vi "motor speed.vi"(0 "IN_A":refnum<k21>="ConnectorA/DIO2", 1 "IN_B":refnum<k21>="ConnectorA/DIO0", 2 "Enable":refnum<k21>="ConnectorA/DIO1", 3 "PWM":refnum<k21>="ConnectorA/DIO8", 4 "speed":i64, 5 "periode":i64, 6 "enable divider":bool, 7 "divider":fxp<+,4,4>, 9 "brake":bool) -> ()   [LabVIEW 2019]
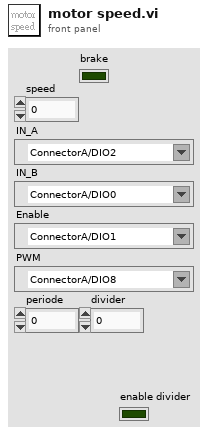
[diagram p1: front panel]
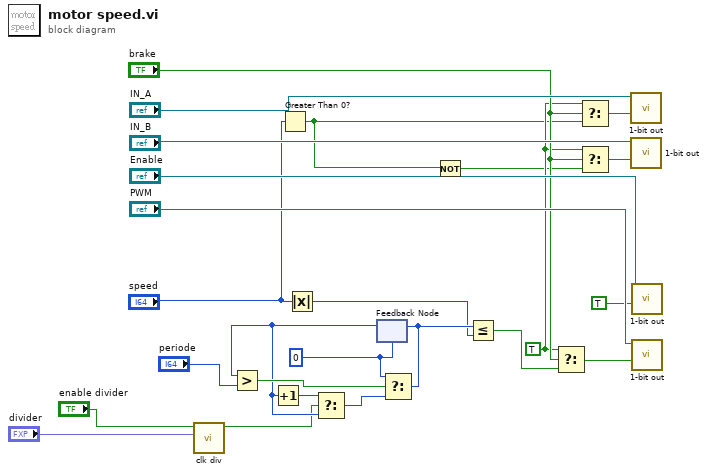
[diagram p0: block diagram]
diagram:
  w3 = TRUE ("t")
  w25 = i64 0
  n1 = call "clk div.vi"("divider"="divider", "enable divider"="enable divider") -> ("f"=w17:bool)  [unwired: 9 in]
  n2 = Greater Than 0?(x="speed") -> (x > 0?=w1:bool)
  n3 = Absolute Value(x="speed") -> (abs(x)=w15:i64)
  n4 = feedback #1(w25) -> (w19:i64)
  n5 = Greater?(x=w19, y="periode") -> (0:w23:bool)
  n6 = Increment(x=w19) -> (x+1=w22:i64)
  n7 = Select(t=w22, s=w17, f=w19) -> (s? t:f=w21:i64)
  n8 = Select(t=w25, s=w23, f=w21) -> (s? t:f=w16:i64)
  n9 = feedback-in #1(w16) -> ()
  n10 = Not(x=w1) -> (.not. x?=w2:bool)
  n11 = Less Or Equal?(x=w16, y=w15) -> (x <= y?=w10:bool)
  n12 = Select(t=w3, s="brake", f=w10) -> (s? t:f=w11:bool)
  n13 = Select(t=w3, s="brake", f=w1) -> (s? t:f=w5:bool)
  n14 = Select(t=w3, s="brake", f=w2) -> (s? t:f=w6:bool)
  n15 = call "1-bit out.vi"("OUT"=w5, "DIO Refnum"="IN_A") -> ()  [unwired: 10 in]
  n16 = call "1-bit out.vi"("OUT"=w6, "DIO Refnum"="IN_B") -> ()  [unwired: 10 in]
  n17 = call "1-bit out.vi"("OUT"=TRUE, "DIO Refnum"="Enable") -> ()  [unwired: 10 in]
  n18 = call "1-bit out.vi"("OUT"=w11, "DIO Refnum"="PWM") -> ()  [unwired: 10 in]
